vi "p2.vi"() -> ()   [LabVIEW 2015]
panel:
  out "Status":bool
  out "Iteration":i32
  out "Current Number":dbl
  in  "Match Numberl":dbl
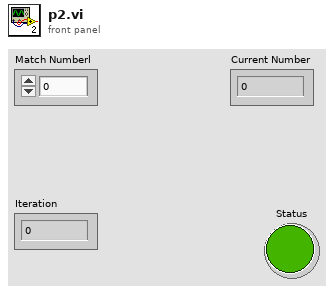
[diagram p1: front panel]
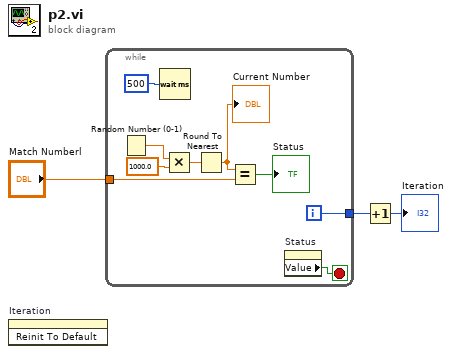
[diagram p0: block diagram]
diagram:
  n1 = invoke on="Iteration" class="DigNum (strict)" method="Reinit To Default"() -> ()  [unwired: 3 in, 3 out]
  n2 = while {
    tunnel: "Match Numberl" -> [w7]
    tunnel: [w6] -> w1
    i -> [w6]
    stop <- w5 stop-if-true
    n3 = Random Number (0-1)() -> (number: 0 to 1=w11:dbl)
    n4 = Wait (ms)(milliseconds to wait=u32 500) -> ()  [unwired: 1 out]
    n5 = Multiply(x=w11, y=1000.0) -> (x*y=w10:dbl)
    n6 = Round To Nearest(number=w10) -> (nearest integer value=w9:dbl)
    "Current Number" <- w9
    n7 = Equal?(x=w9, y=w7) -> (x = y?=→"Status":bool)
    n8 = property on="Status" class="Bool (strict)"() -> ("Value"=w5:bool)  [unwired: 2 in, 2 out]
  }
  n9 = Increment(x=w1) -> (x+1=→"Iteration":i32)
